vi "string function2.vi"() -> ()   [LabVIEW 2019]
panel:
  out "all upper case":string
  out "all upper case":string
  in  "string 1":string="happy"
  in  "string 2":string="birthday"
  out "all lower case":string
  in  "string 3":string="to you!!"
  out "Substring":string="\"Happy mothers day !!! \n t"
  in  "String 1":string="\"Happy mothers day !!! \n to the best mom in the world....\" #youinspireme\n"
  # "STRING FUNCTION"
  # "3) String subset function"
  # "4) String upper case and lower case"
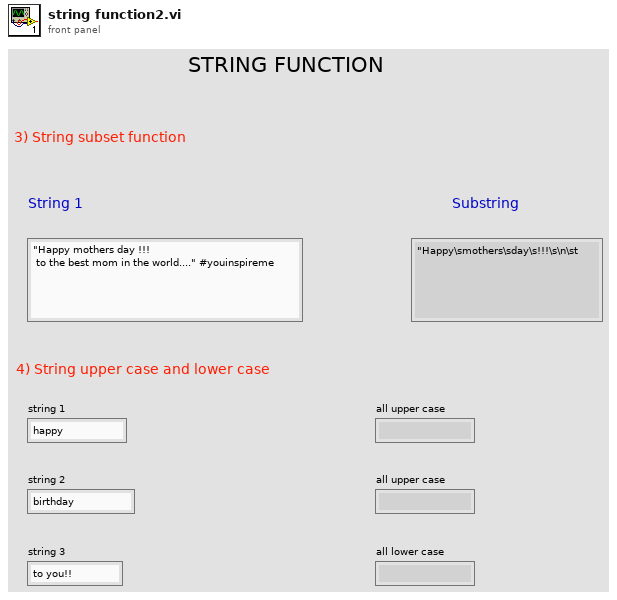
[diagram p1: front panel]
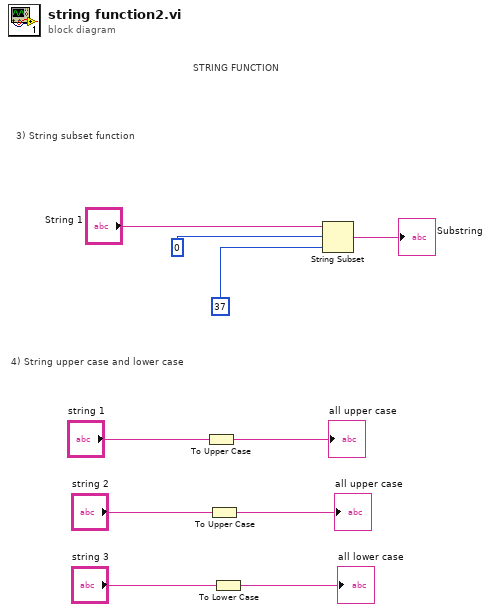
[diagram p0: block diagram]
diagram:
  # "4) String upper case and lower case"
  # "3) String subset function"
  # "STRING FUNCTION"
  n1 = To Upper Case(1:"string 1") -> (0:→"all upper case":string)
  n2 = To Upper Case(1:"string 2") -> (0:→"all upper case":string)
  n3 = To Lower Case(string="string 3") -> (all lower case string=→"all lower case":string)
  n4 = String Subset(string="String 1", offset (0)=0, length (rest)=37) -> (substring=→"Substring":string)
